vi "Output Motor Enable Bits.vi"   [LabVIEW 2009]
uses:
  Motor Control Global.vi
  Motor Output Global.vi
  <vilib>/eio/EIONode/EIONode.xnode
  <vilib>/rvi/eio/nirviEIOImplementation/nirviEIOImplementation.xnode
  <vilib>/rvi/eio/common/nirviEmuTemplateMethod_noerrors.vi
  <vilib>/rvi/eio/common/nirviEmuClasses.ctl
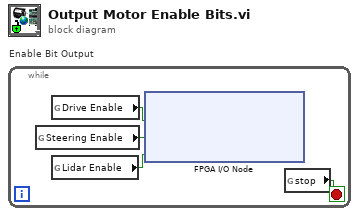
[diagram p0: block diagram]
diagram:
  n1 = while "Enable Bit Output" {
    stop <- w4 stop-if-true
    n2 = global read "Motor Output Global.vi" "Steering Enable"() -> (w2:bool)
    n3 = global read "Motor Output Global.vi" "Drive Enable"() -> (w3:bool)
    n4 = global read "Motor Output Global.vi" "Lidar Enable"() -> (w1:bool)
    n5 = xnode "FPGA I/O Node"("Drive Motor Enable"=w3, "Steering Motor Inhibit"=w2, "Lidar Motor Inhibit"=w1) -> ()  [unwired: 3 in, 3 out]
    n6 = global read "Motor Control Global.vi" "stop"() -> (w4:bool)
  }
